vi "DFD Load NStage MRate Filter from Text File.vi"(8 "error in (no error)":errorcluster, 10 "file path in":path) -> (0 "error out":errorcluster, 2 "file path out":path, 3 "multirate filters out":T1[](array[typedef]) {"mMRate_SumWl" min=1 max=32 step=1; "mMRate_InputIwl" min=1 max=32 step=1; "mMRate_GainWl" min=1 max=32 step=1; "mMRate_OutputWl" min=1 max=32 step=1; "mMRate_InputWl" min=1 max=32 step=1; "mMRate_CoefWl" min=1 max=32 step=1; "mMRate_Mode" items=["Default"=-1, "No Rate Change"=0, "Interpolation"=1, "Decimation"=2, "Interpolated"=3, "Rational"=4]})   [LabVIEW 2017, in "NI_DigFilterLicensed.lvlib"]
doc: "Retrieves a filter or a filter bank from a text file in XML format. You must manually select the polymorphic instance you want to use."
uses:
  <vilib>/addons/Digital Filter Design/NI_DigFilterLicensed.lvlib
  <vilib>/addons/Digital Filter Design/_Objects.llb/DFD Multirate Filter Obj.ctl
  <vilib>/addons/Digital Filter Design/_Objects.llb/DFD Multirate Mode.ctl
  <vilib>/addons/Digital Filter Design/_Objects.llb/DFD Coef Norm Type.ctl
  <vilib>/addons/Digital Filter Design/_Objects.llb/DFD Round-off Mode.ctl
  <vilib>/addons/Digital Filter Design/_Objects.llb/DFD FXP MRate Multiply Mode.ctl
  <vilib>/addons/Digital Filter Design/NI_DigFilter_Process.lvlib
panel:
  in  "multirate filter":T1={"mMRate_Structure"=enum."FIR", "mMRate_Mode"=0, "mMRate_Factor"=1, "mMRate_FIRParams"={"mMRate_FIR_H"=[], "mMRate_FIR_IsNyquist?"=FALSE, "mMRate_FIR_IsSymmetric?"=FALSE}, "mMRate_CICParams"={"mMRate_CIC_#Stage"=2, "mMRate_CIC_Lag"=1, "mMRate_CIC_Type"=enum."Lowpass"}, "mMRate_Order"=0, "mMRate_Version"="2.0", "mMRate_Comments"="", "mMRate_RationalFactor"={"mMRate_L"=-1, "mMRate_M"=-1}, "mMRate_Fs"=1.0, "mMRate_Quantized?"=FALSE, "mMRate_QFilterGain"=1.0, "mMRate_CoefWl"=16, "mMRate_Scaling"={"mMRate_ScaleByPowerOf2?"=FALSE, "mMRate_ScaleType"=enum."Time Domain 1-Norm"}, "mMRate_InputWl"=16, "mMRate_OutputWl"=16, "mMRate_OutputMode"=enum."Nearest", "mMRate_MultMode"=enum."Truncated", "mMRate_BitPruning"=FALSE, "mMRate_GainWl"=16, "mMRate_OutputFwl"=0, "mMRate_SumIwl"=0, "mMRate_InputIwl "=16, "mMRate_SumWl"=32, "mMRate_CoefIwl"=0} {"mMRate_SumWl" min=1 max=32 step=1; "mMRate_InputIwl" min=1 max=32 step=1; "mMRate_GainWl" min=1 max=32 step=1; "mMRate_OutputWl" min=1 max=32 step=1; "mMRate_InputWl" min=1 max=32 step=1; "mMRate_CoefWl" min=1 max=32 step=1; "mMRate_Mode" items=["Default"=-1, "No Rate Change"=0, "Interpolation"=1, "Decimation"=2, "Interpolated"=3, "Rational"=4]}
  in  "multirate filters in":T1[](array[typedef]) {"mMRate_SumWl" min=1 max=32 step=1; "mMRate_InputIwl" min=1 max=32 step=1; "mMRate_GainWl" min=1 max=32 step=1; "mMRate_OutputWl" min=1 max=32 step=1; "mMRate_InputWl" min=1 max=32 step=1; "mMRate_CoefWl" min=1 max=32 step=1; "mMRate_Mode" items=["Default"=-1, "No Rate Change"=0, "Interpolation"=1, "Decimation"=2, "Interpolated"=3, "Rational"=4]}
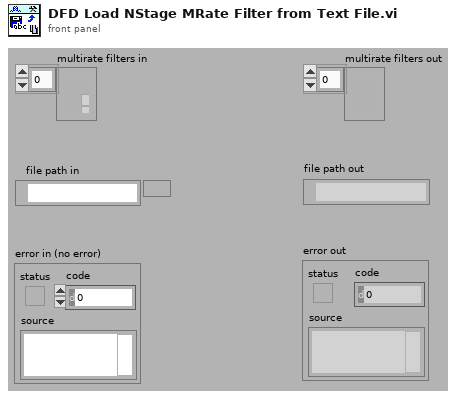
[diagram p1: front panel]
types:
  T1 = typedef "NI_DigFilterLicensed.lvlib/DFD Multirate Filter Obj.ctl" = cluster{"mMRate_Structure":enum16{"CIC", "FIR", "IIR", "Lattice"}, "mMRate_Mode":T2, "mMRate_Factor":i32, "mMRate_FIRParams":cluster{"mMRate_FIR_H":dbl[], "mMRate_FIR_IsNyquist?":bool, "mMRate_FIR_IsSymmetric?":bool}, "mMRate_CICParams":cluster{"mMRate_CIC_#Stage":i32, "mMRate_CIC_Lag":i32, "mMRate_CIC_Type":enum16{"Lowpass", "Highpass"}}, "mMRate_Order":i32, "mMRate_Version":string, "mMRate_Comments":string, "mMRate_RationalFactor":cluster{"mMRate_L":i32, "mMRate_M":i32}, "mMRate_Fs":dbl, "mMRate_Quantized?":bool, "mMRate_QFilterGain":dbl, "mMRate_CoefWl":i16, "mMRate_Scaling":cluster{"mMRate_ScaleByPowerOf2?":bool, "mMRate_ScaleType":T3}, "mMRate_InputWl":i16, "mMRate_OutputWl":i16, "mMRate_OutputMode":T4, "mMRate_MultMode":T5, "mMRate_BitPruning":bool, "mMRate_GainWl":i16, "mMRate_OutputFwl":i16, "mMRate_SumIwl":i16, "mMRate_InputIwl ":i16, "mMRate_SumWl":i16, "mMRate_CoefIwl":i16}
  T2 = typedef "NI_DigFilterLicensed.lvlib/DFD Multirate Mode.ctl" = i16
  T3 = typedef "NI_DigFilterLicensed.lvlib/DFD Coef Norm Type.ctl" = enum16{"No Norm", "Time Domain 1-Norm", "Time Domain 2-Norm", "Time Domain Inf-Norm"}
  T4 = typedef "NI_DigFilterLicensed.lvlib/DFD Round-off Mode.ctl" = enum16{"Nearest", "Truncation"}
  T5 = typedef "NI_DigFilterLicensed.lvlib/DFD FXP MRate Multiply Mode.ctl" = enum16{"Truncated", "Full"}
  T6 = enum16{"open", "open or create", "create or replace", "create", "open (read only)"}
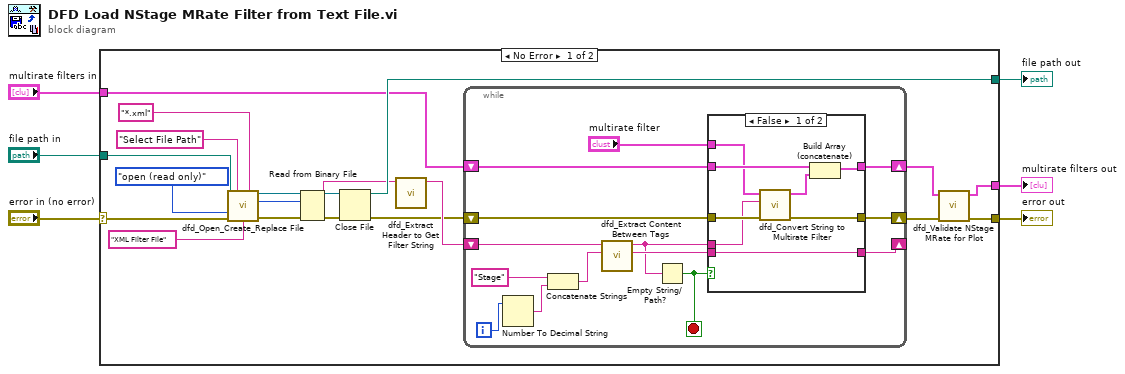
[diagram p0: block diagram]
diagram:
  n1 = case shown="No Error" "error in (no error)" {
    selector: "error in (no error)" -> [w23 w53]
    tunnel: [w9 w53] -> w5
    tunnel: "file path in" -> [w26 w52]
    tunnel: [w16 w52] -> w3
    tunnel: "multirate filters in" -> [w11 _]
    tunnel: [w7 _] -> w1
    frame No Error {
      n2 = call <vilib>:"dfd_Open_Create_Replace File.vi"("file path"=w26, "prompt"="Select File Path" ("Prompt"), "pattern"="*.xml", "function (open:0)"=T6."open (read only)", "error in (no error)"=w23, "pattern label"="XML Filter File") -> ("refnum"=w22:refnum<file>, "file size (bytes)"=w19:i32, "error out"=w24:errorcluster)  [unwired: 2 in, 5 out]
      n3 = Read from Binary File(8:w24, 10:w19, 11:w22) -> (0:w18:errorcluster, 2:w15:string, 3:w17:refnum<file>)  [unwired: 4 out]
      n4 = Close File(refnum=w17, error in=w18) -> (path=w16:path, error out=w12:errorcluster)
      n5 = call <vilib>:"dfd_Extract Header to Get Filter String.vi"("string in"=w15) -> ("string out"=w13:string)  [unwired: 10 out]
      n6 = while {
        shift-right: [w39] -> w10
        shift-left: w12 -> [w40]
        shift-right: [w31] -> _
        shift-left: w13 -> [w33]
        shift-right: [w28] -> w8
        shift-left: w11 -> [w38]
        i -> [w36]
        stop <- w29 stop-if-true
        n7 = Number To Decimal String(number=w36) -> (decimal integer string=w35:string)  [unwired: 1 out]
        n8 = Concatenate Strings("Stage" ("string"), w35) -> (w34:string)
        n9 = call <vilib>:"dfd_Extract Content Between Tags.vi"("element"=w34, "xml string with tag"=w33) -> ("remaining string"=w32:string, "content"=w30:string)  [unwired: 8 out]
        n10 = Empty String/Path?(string/path=w30) -> (empty?=w29:bool)
        n11 = case shown="False" w29 {
          tunnel: w40 -> [w48 w51]
          tunnel: [w47 w51] -> w39
          tunnel: w38 -> [w44 w49]
          tunnel: w30 -> [w46 _]
          tunnel: [w45 w50] -> w31
          tunnel: w32 -> [w45 w50]
          tunnel: "multirate filter" -> [w41 _]
          tunnel: [w42 w49] -> w28
          frame False {
            n12 = call <vilib>:"dfd_Convert String to Multirate Filter.vi"("error in (no error)"=w48, "xml string"=w46, "multirate filter in"=w41) -> ("error out"=w47:errorcluster, "multirate filter out"=w43:T1)  [unwired: 7 out]
            n13 = Build Array (concatenate)(w44, w43) -> (w42:T1[])
          }
          frame True {
          }
        }
      }
      n14 = call <vilib>:"dfd_Validate NStage MRate for Plot.vi"("error in (no error)"=w10, "multirate filters in"=w8) -> ("error out"=w9:errorcluster, "multirate filters out"=w7:T1[])  [unwired: 8 out]
    }
    frame Error {
    }
  }
  "error out" <- w5
  "file path out" <- w3
  "multirate filters out" <- w1
